vi "checkPNhistory.vi"(10 "PN":string, 11 "Path":path) -> (3 "Array":string[][](array[string]))   [LabVIEW 2020]
uses:
  <vilib>/Utility/error.llb/whitespace.ctl
  <vilib>/Utility/config.llb/Read Key (String).vi
  <vilib>/Utility/config.llb/NI_LVConfig.lvlib
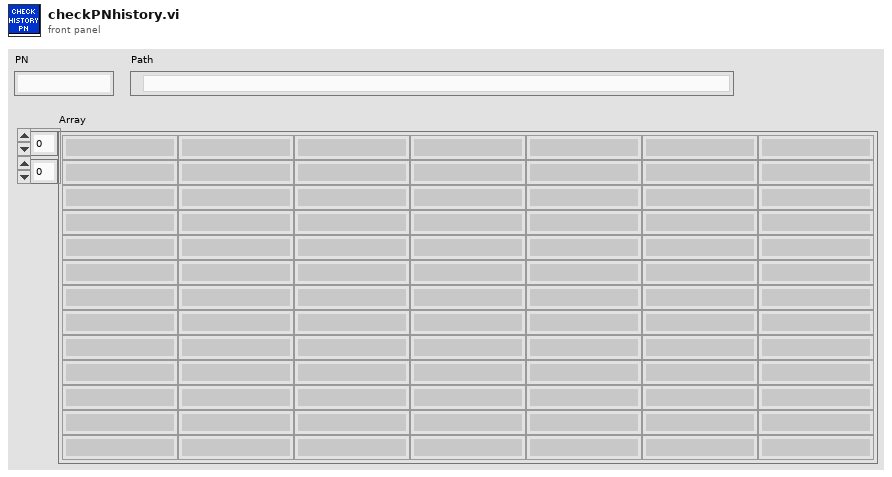
[diagram p1: front panel]
types:
  T1 = typedef "NI_LVConfig.lvlib/Config Data RefNum.ctl" = refnum<k1>
  T2 = typedef "whitespace.ctl" = u16
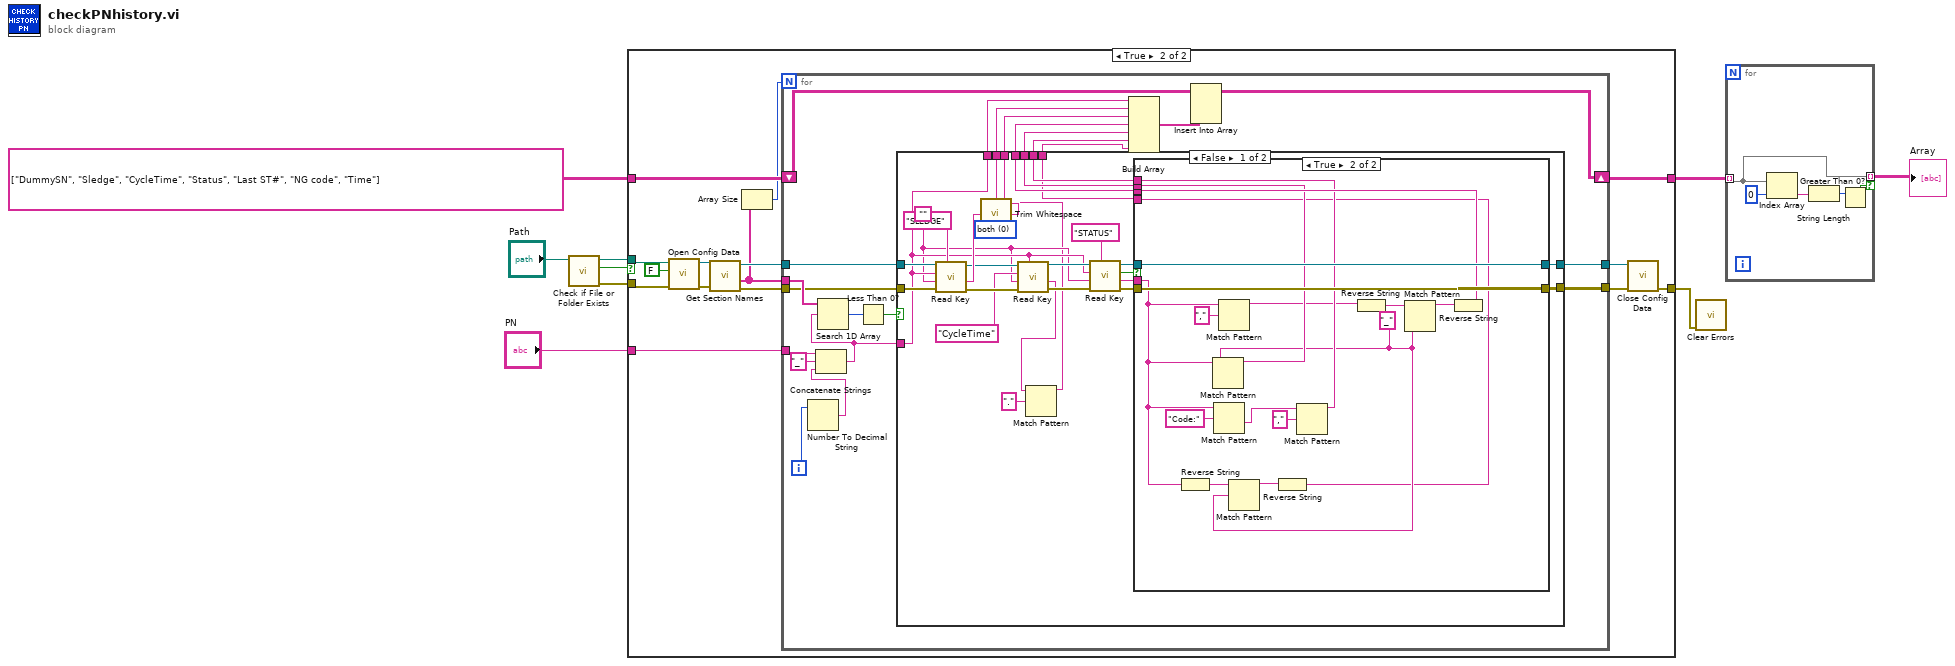
[diagram p0: block diagram]
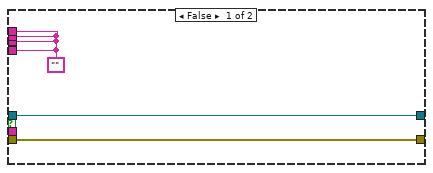
[diagram p3: hidden frame]
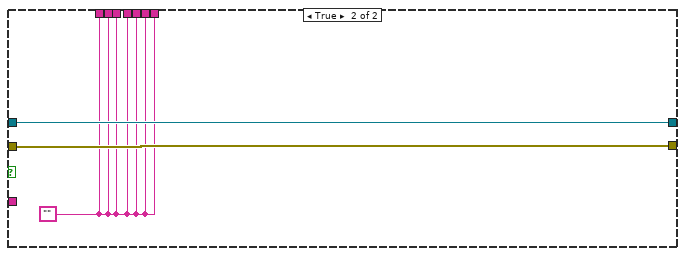
[diagram p4: hidden frame]
diagram:
  n1 = call <vilib>:"Check if File or Folder Exists.vi"("path"="Path") -> ("error out"=w5:errorcluster, "file or folder exists?"=w8:bool, "dup path"=w6:path)  [unwired: 8 in]
  n2 = case shown="True" w8 {
    tunnel: string[][] [["DummySN", "Sledge", "CycleTime", "Status", "Last ST#", "NG code", "Time"]] -> [w11 w18]
    tunnel: [w11 w19] -> w3
    tunnel: w6 -> [_ w25]
    tunnel: w5 -> [w10 w26]
    tunnel: "PN" -> [_ w15]
    tunnel: [w10 w12] -> w1
    frame False {
    }
    frame True {
      n3 = call <vilib>:"Open Config Data.vi"("error in (no error)"=w26, "create file if necessary (T)"=FALSE, "configuration file path"=w25) -> ("error out"=w23:errorcluster, "refnum"=w22:T1)  [unwired: 6 in, 1 out]
      n4 = call <vilib>:"Get Section Names.vi"("error in (no error)"=w23, "refnum"=w22) -> ("error out"=w21:errorcluster, "section names"=w17:string[], "refnum out"=w20:T1)  [unwired: 7 in]
      n5 = Array Size(array=w17) -> (size(s)=w16:i32)
      n6 = for {
        N: w16 -> [_]
        tunnel: w17 -> [w44]
        tunnel: w21 -> [w34]
        tunnel: w20 -> [w33]
        shift-right: [w48] -> w19
        shift-left: w18 -> [w47]
        tunnel: w15 -> [w46]
        tunnel: [w32] -> w14
        tunnel: [w31] -> w13
        i -> [w45]
        n7 = Number To Decimal String(number=w45) -> (decimal integer string=w30:string)  [unwired: 1 in]
        n8 = Concatenate Strings(w46, "_" ("string"), w30) -> (w35:string)
        n9 = Search 1D Array(1D array=w44, element=w35) -> (index of element=w42:i32)  [unwired: 1 in]
        n10 = Less Than 0?(x=w42) -> (x < 0?=w41:bool)
        n11 = case shown="False" w41 {
          tunnel: [w64 w96] -> w40
          tunnel: [w55 w96] -> w39
          tunnel: [w56 w96] -> w38
          tunnel: [w49 w96] -> w37
          tunnel: [w71 w96] -> w36
          tunnel: w35 -> [w64 _]
          tunnel: w34 -> [w75 w98]
          tunnel: w33 -> [w74 w97]
          tunnel: [w59 w98] -> w32
          tunnel: [w57 w97] -> w31
          tunnel: [w53 w96] -> w28
          tunnel: [w52 w96] -> w27
          frame False {
            w70 = T2 0 items=["both", "start of string", "end of string"] ("location (both)")
            w62 = ""
            n12 = call-poly <vilib>:"Read Key.vi"("section"="SLEDGE", "error in (no error)"=w75, "default value"=w62, "key"=w64, "refnum"=w74) -> ("error out"=w69:errorcluster, "value"=w72:string, "refnum out"=w68:T1)  [unwired: 3 in, 1 out]
            n13 = call <vilib>:"Trim Whitespace.vi"("string"=w72, "location (both)"=w70) -> ("trimmed string"=w71:string)
            n14 = call-poly <vilib>:"Read Key.vi"("section"=w64, "error in (no error)"=w69, "default value"=w62, "key"="CycleTime", "refnum"=w68) -> ("error out"=w66:errorcluster, "value"=w51:string, "refnum out"=w65:T1)  [unwired: 3 in, 1 out]
            n15 = Match Pattern(string=w51, regular expression=".") -> (before substring=w49:string)  [unwired: 1 in, 3 out]
            n16 = call-poly <vilib>:"Read Key.vi"("section"="STATUS", "error in (no error)"=w66, "default value"=w62, "key"=w64, "refnum"=w65) -> ("error out"=w60:errorcluster, "value"=w54:string, "found?"=w61:bool, "refnum out"=w58:T1)  [unwired: 3 in]
            n17 = case shown="True" w61 {
              tunnel: w60 -> [w78 w95]
              tunnel: [w78 w95] -> w59
              tunnel: w58 -> [w77 w94]
              tunnel: [w77 w94] -> w57
              tunnel: [w76 w91] -> w56
              tunnel: [w76 w90] -> w55
              tunnel: [w76 w86] -> w53
              tunnel: w54 -> [_ w80]
              tunnel: [w76 w79] -> w52
              frame False {
                w76 = ""
              }
              frame True {
                w81 = "_" ("regular expression")
                n18 = Reverse String(1:w80) -> (0:w83:string)
                n19 = Match Pattern(string=w80, regular expression=w81) -> (before substring=w90:string)  [unwired: 1 in, 3 out]
                n20 = Match Pattern(string=w80, regular expression="Code:") -> (after substring=w87:string)  [unwired: 1 in, 3 out]
                n21 = Match Pattern(string=w80, regular expression=",") -> (before substring=w84:string)  [unwired: 1 in, 3 out]
                n22 = Match Pattern(string=w83, regular expression=w81) -> (before substring=w82:string)  [unwired: 1 in, 3 out]
                n23 = Reverse String(1:w82) -> (0:w79:string)
                n24 = Match Pattern(string=w87, regular expression=",") -> (before substring=w86:string)  [unwired: 1 in, 3 out]
                n25 = Reverse String(1:w84) -> (0:w93:string)
                n26 = Match Pattern(string=w93, regular expression=w81) -> (before substring=w92:string)  [unwired: 1 in, 3 out]
                n27 = Reverse String(1:w92) -> (0:w91:string)
              }
            }
          }
          frame True {
            w96 = ""
          }
        }
        n28 = Build Array(w40, w36, w37, w38, w39, w28, w27) -> (w43:string[])
        n29 = Insert Into Array(array=w47, new element=w43) -> (w48:string[][])  [unwired: 2 in]
      }
      n30 = call <vilib>:"Close Config Data.vi"("error in (no error)"=w14, "refnum"=w13) -> ("error out"=w12:errorcluster)  [unwired: 8 in, 1 out]
    }
  }
  n31 = call <vilib>:"Clear Errors.vi"("error in (no error)"=w1) -> ()  [unwired: 5 in, 2 out]
  n32 = for {
    tunnel: w3 -> [w102] mode=indexing
    tunnel: [w102] -> w2 mode=indexing if=w99
    n33 = Index Array(array=w102, index=0) -> (element=w101:string)
    n34 = String Length(string=w101) -> (length=w100:i32)
    n35 = Greater Than 0?(x=w100) -> (x > 0?=w99:bool)
  }
  "Array" <- w2
